vi "Position Numeric Below Button.vi"(8 "error in (no error)":errorcluster, 10 "Button Ref":refnum<vi>, 11 "Aircraft Id Ref":refnum<vi>) -> (0 "error out":errorcluster)   [LabVIEW 2014]
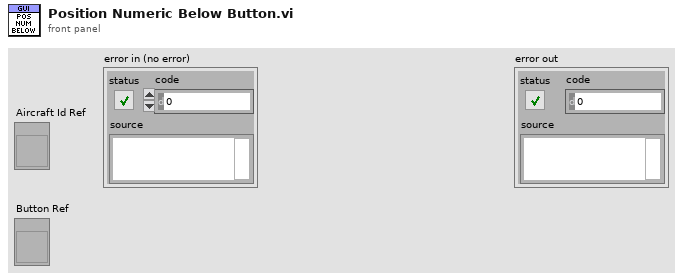
[diagram p1: front panel]
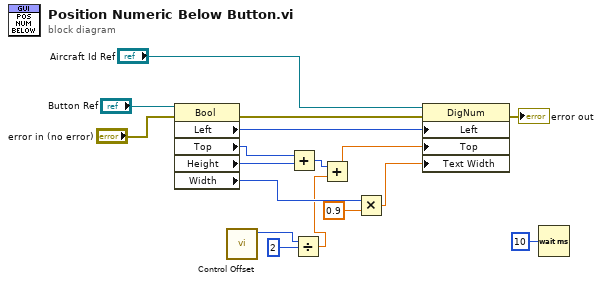
[diagram p0: block diagram]
diagram:
  n1 = property class="Bool"(reference="Button Ref", error in="error in (no error)") -> (error out=w14:errorcluster, "Left"=w15:i32, "Top"=w13:i32, "Height"=w12:u32, "Width"=w7:u32)  [unwired: 1 out]
  n2 = call "Control Offset.vi"() -> ("Offset From Tab Edge in (px)"=w4:i32)  [unwired: 11 in]
  n3 = Add(x=w13, y=w12) -> (x+y=w11:u32)
  n4 = Divide(x=w4, y=2) -> (x/y=w2:dbl)
  n5 = Add(x=w11, y=w2) -> (x+y=w10:dbl)
  n6 = Multiply(x=w7, y=0.9) -> (x*y=w5:dbl)
  n7 = property class="DigNum"(reference="Aircraft Id Ref", error in=w14, "Left"=w15, "Top"=w10, "Text Width"=w5) -> (error out=→"error out":errorcluster)  [unwired: 1 out]
  n8 = Wait (ms)(milliseconds to wait=u32 10) -> ()  [unwired: 1 out]
